vi "debugger read current config.vi"() -> (1 "VI List":string[](array[string]), 2 "Current Config":T1)   [LabVIEW 2011]
uses:
  ITK EXT/utils/keyedarr.llb/Keyed Array.ctl
  ITK EXT/utils/strutil.llb/Case Matching.ctl
  server/server lib/Spartan Version.vi
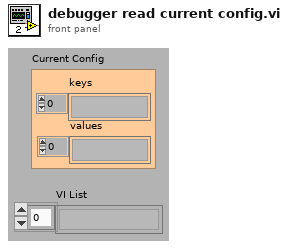
[diagram p1: front panel]
types:
  T1 = typedef "Keyed Array.ctl" = cluster{"keys":string[], "values":string[]}
  T2 = cluster{"webserver.rootpath":path, "server.tcp.enabled":bool, "server.tcp.port":u32, "server.tcp.access":string[], "server.vi.access":string[], "webserver.enabled":bool, "webserver.port":u16, "webserver.logenabled":bool, "webserver.logpath":path}
  T3 = typedef "OGAB Version.ctl" = cluster{"Version":string, "Build Number":u32, "Build Date/Time":dbl}
  T4 = typedef "Case Matching.ctl" = enum16{"a != A", "a == A", "system"}
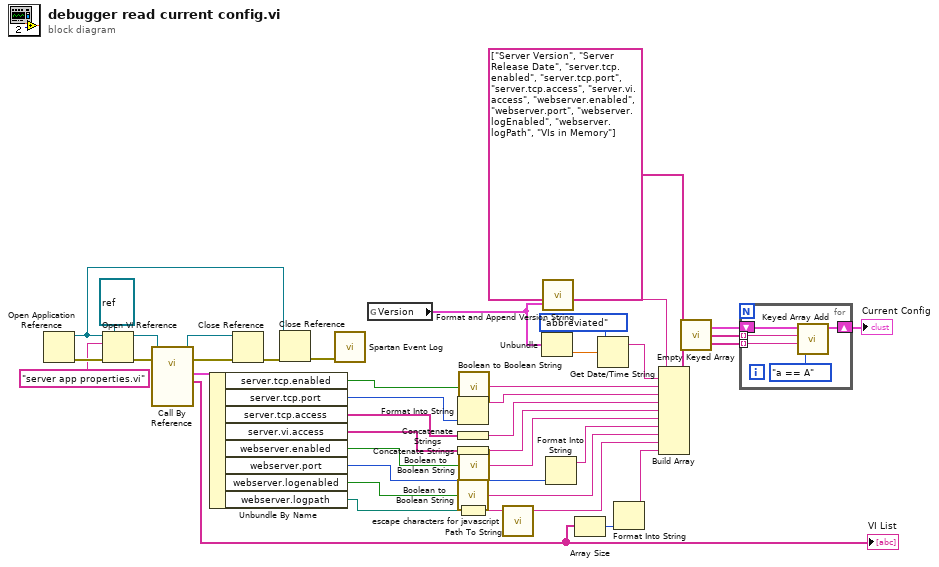
[diagram p0: block diagram]
diagram:
  n1 = Open Application Reference() -> (0:w20:errorcluster, 3:w13:refnum<vi>)  [unwired: 4 in]
  n2 = Open VI Reference(type specifier VI Refnum (for type only)=refnum<vi> refnum, application reference (local)=w13, vi path="server app properties.vi", error in (no error)=w20) -> (vi reference=w18:refnum<vi>, error out=w19:errorcluster)  [unwired: 2 in]
  n3 = call-by-ref "?"(reference=w18, error in=w19) -> (reference out=w15:refnum<vi>, error out=w16:errorcluster, "App.AllVIs"=w11:string[], "App.Properties"=w10:T2)  [unwired: 9 in, 1 out]
  "VI List" <- w11
  n4 = Unbundle By Name(w10) -> ("server.tcp.enabled"=w9:bool, "server.tcp.port"=w8:u32, "server.tcp.access"=w7:string[], "server.vi.access"=w6:string[], "webserver.enabled"=w5:bool, "webserver.port"=w4:u16, "webserver.logenabled"=w3:bool, "webserver.logpath"=w2:path)
  n5 = Close Reference(reference=w15, error in (no error)=w16) -> (error out=w14:errorcluster)
  n6 = Close Reference(reference=w13, error in (no error)=w14) -> (error out=w12:errorcluster)
  n7 = call "Spartan Event Log.vi"("error in (no error)"=w12) -> ()  [unwired: 7 in, 1 out]
  n8 = global read "Spartan Version.vi" "Version"() -> (w21:T3)
  n9 = Format Into String(w8) -> (resulting string=w29:string)  [unwired: 3 in, 1 out]
  n10 = Concatenate Strings(w7) -> (w33:string)
  n11 = Concatenate Strings(w6) -> (w32:string)
  n12 = call "Boolean to Boolean String.vi"("Boolean"=w3) -> ("Boolean string"=w24:string)  [unwired: 1 in]
  n13 = Path To String(path=w2) -> (string=w26:string)
  n14 = call "Boolean to Boolean String.vi"("Boolean"=w9) -> ("Boolean string"=w30:string)  [unwired: 1 in]
  n15 = call "Boolean to Boolean String.vi"("Boolean"=w5) -> ("Boolean string"=w28:string)  [unwired: 1 in]
  n16 = call "escape characters for javascript.vi"("String (\"\")"=w26) -> ("escaped String"=w25:string)  [unwired: 4 in]
  n17 = Unbundle(w21) -> ("Build Date/Time"=w40:dbl)  [unwired: 2 out]
  n18 = call "Format and Append Version String.vi"("Version"=w21) -> ("String with Version"=w36:string)  [unwired: 1 in, 9 out]
  n19 = Format Into String(w4) -> (resulting string=w27:string)  [unwired: 3 in, 1 out]
  n20 = Array Size(array=w11) -> (size(s)=w37:i32)
  n21 = Get Date/Time String(date format (0)=enum16{"short", "long", "abbreviated"}."abbreviated", seconds (now)=w40) -> (date string=w35:string)  [unwired: 2 out]
  n22 = Format Into String(w37) -> (resulting string=w31:string)  [unwired: 3 in, 1 out]
  n23 = Build Array(w36, w35, w30, w29, w33, w32, w28, w27, w24, w25, w31) -> (w34:string[])
  n24 = call "Empty Keyed Array.vi"() -> ("empty keyed array"=w23:T1)  [unwired: 3 in]
  n25 = for {
    shift-right: [w43] -> w22
    shift-left: w23 -> [w45]
    tunnel: string[] ["Server Version", "Server Release Date", "server.tcp.enabled", "server.tcp.port", "server.tcp.access", "server.vi.access", "webserver.enabled", "webserver.port", "webserver.logEnabled", "webserver.logPath", "VIs in Memory"] -> [w42] mode=indexing
    tunnel: w34 -> [w41] mode=indexing
    n26 = call "Keyed Array Add.vi"("case matching (sensitive)"=Case_Matching."a == A", "value"=w41, "key"=w42, "array in"=w45) -> ("array out"=w43:T1)  [unwired: 3 out]
  }
  "Current Config" <- w22
